vi "ma_Locate three fingers.vi"   [LabVIEW 2020, in "NI_MAPro.lvlib"]
uses:
  NI_MAPro.lvlib
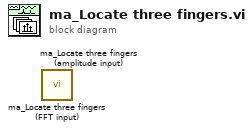
[diagram p0: block diagram]
diagram:
  n1 = call "ma_Locate three fingers (FFT input).vi"() -> ()  [unwired: 4 in, 2 out]
  n2 = call "ma_Locate three fingers (amplitude input).vi"() -> ()  [unwired: 4 in, 2 out]
